vi "WS104x_NI_6501_Cntrl RF Switch.vi"(0 "SW1":bool=TRUE, 1 "NI-6051":T1={"Addr Cntrl 1"="Dev1/port0/line0", "Addr Cntrl 2"="Dev1/port0/line1", "Addr Cntrl 3"="Dev1/port0/line2", "Addr Cntrl 4"="Dev1/port0/line3"}, 5 "SW2":bool, 7 "SW3":bool, 9 "SW4":bool, 11 "error in":errorcluster) -> (15 "error out":errorcluster)   [LabVIEW 2012]
doc: "I. Description:\nThis example demonstrates how to write values to a digital output channel.\n\nII. Instructions for Running:\n1. Select the digital lines on the DAQ device to be written.\n2. Select a value to write.\nNote: The array control is sized for 8 lines, if using a different amount of lines, change the number of elements in the array to equal the number of lines chosen.\n\nIII. Block Diagram Steps:\n1. Create a Digital Output channel. Use one channel for all lines. You can alternatively use one channel for each line, but then use a different polymorphic version of the DAQmx Write VI.\n2. Call the Start VI to start the task.\n3. Write the digital Boolean array data in a loop until the user hits the stop button or an error occurs. This write VI writes a single sample of digital data on demand, so no timeout is necessary.\n4. Call the Clear Task VI to clear the Task.\n5. Use the popup dialog box to display an error or warning if any.\n\nIV. I/O Connections Overview:\nMake sure your signal output terminals match the Lines I/O Control. In this case wire the item to receive the signal to the first eight digital lines on your DAQ Device."
uses:
  <vilib>/DAQmx/create/channels.llb/DAQmx Create Channel (DO-Digital Output).vi
  <vilib>/DAQmx/write.llb/DAQmx Write (Digital Bool 1Line 1Point).vi
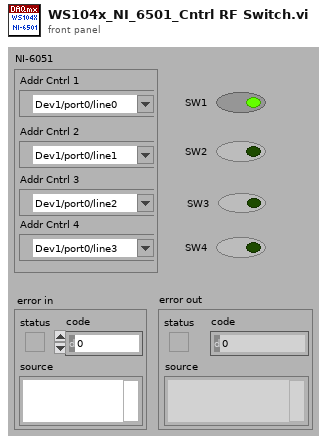
[diagram p1: front panel]
types:
  T1 = cluster{"Addr Cntrl 1":tag, "Addr Cntrl 2":tag, "Addr Cntrl 3":tag, "Addr Cntrl 4":tag}
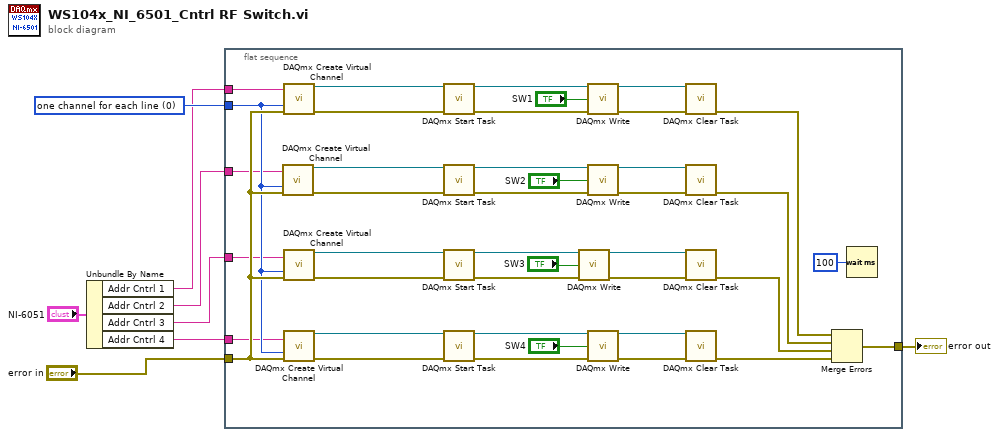
[diagram p0: block diagram]
diagram:
  w5 = 0 items=["one channel for each line", "one channel for all lines"] ("line grouping")
  n1 = Unbundle By Name("NI-6051") -> ("Addr Cntrl 1"=w4:tag, "Addr Cntrl 2"=w3:tag, "Addr Cntrl 3"=w2:tag, "Addr Cntrl 4"=w1:tag)
  n2 = flat-sequence {
    tunnel: "error in" -> [w20]
    tunnel: [w15] -> w7
    tunnel: w5 -> [w13]
    tunnel: w4 -> [w12]
    tunnel: w3 -> [w11]
    tunnel: w2 -> [w10]
    tunnel: w1 -> [w9]
    frame #0 {
      n3 = call-poly <vilib>:"DAQmx Create Virtual Channel.vi"("lines"=w11, "line grouping"=w13, "error in"=w20) -> ("task out"=w39:refnum<k21>, "error out"=w40:errorcluster)  [unwired: 11 in]
      n4 = call-poly <vilib>:"DAQmx Create Virtual Channel.vi"("lines"=w12, "line grouping"=w13, "error in"=w20) -> ("task out"=w44:refnum<k21>, "error out"=w43:errorcluster)  [unwired: 11 in]
      n5 = call-poly <vilib>:"DAQmx Create Virtual Channel.vi"("lines"=w10, "line grouping"=w13, "error in"=w20) -> ("task out"=w30:refnum<k21>, "error out"=w29:errorcluster)  [unwired: 11 in]
      n6 = call-poly <vilib>:"DAQmx Create Virtual Channel.vi"("lines"=w9, "line grouping"=w13, "error in"=w20) -> ("task out"=w25:refnum<k21>, "error out"=w26:errorcluster)  [unwired: 11 in]
      n7 = call <vilib>:"DAQmx Start Task.vi"("task/channels in"=w44, "error in"=w43) -> ("task out"=w46:refnum<k21>, "error out"=w48:errorcluster)  [unwired: 12 in]
      n8 = call <vilib>:"DAQmx Start Task.vi"("task/channels in"=w39, "error in"=w40) -> ("task out"=w37:refnum<k21>, "error out"=w35:errorcluster)  [unwired: 12 in]
      n9 = call <vilib>:"DAQmx Start Task.vi"("task/channels in"=w30, "error in"=w29) -> ("task out"=w32:refnum<k21>, "error out"=w34:errorcluster)  [unwired: 12 in]
      n10 = call <vilib>:"DAQmx Start Task.vi"("task/channels in"=w25, "error in"=w26) -> ("task out"=w23:refnum<k21>, "error out"=w21:errorcluster)  [unwired: 12 in]
      n11 = call-poly <vilib>:"DAQmx Write.vi"("task/channels in"=w32, "data"="SW3", "error in"=w34) -> ("task out"=w31:refnum<k21>, "error out"=w33:errorcluster)  [unwired: 10 in, 1 out]
      n12 = call-poly <vilib>:"DAQmx Write.vi"("task/channels in"=w46, "data"="SW1", "error in"=w48) -> ("task out"=w45:refnum<k21>, "error out"=w47:errorcluster)  [unwired: 10 in, 1 out]
      n13 = call-poly <vilib>:"DAQmx Write.vi"("task/channels in"=w37, "data"="SW2", "error in"=w35) -> ("task out"=w38:refnum<k21>, "error out"=w36:errorcluster)  [unwired: 10 in, 1 out]
      n14 = call-poly <vilib>:"DAQmx Write.vi"("task/channels in"=w23, "data"="SW4", "error in"=w21) -> ("task out"=w24:refnum<k21>, "error out"=w22:errorcluster)  [unwired: 10 in, 1 out]
      n15 = call <vilib>:"DAQmx Clear Task.vi"("task in"=w45, "error in"=w47) -> ("error out"=w19:errorcluster)  [unwired: 13 in]
      n16 = call <vilib>:"DAQmx Clear Task.vi"("task in"=w38, "error in"=w36) -> ("error out"=w18:errorcluster)  [unwired: 13 in]
      n17 = call <vilib>:"DAQmx Clear Task.vi"("task in"=w31, "error in"=w33) -> ("error out"=w17:errorcluster)  [unwired: 13 in]
      n18 = call <vilib>:"DAQmx Clear Task.vi"("task in"=w24, "error in"=w22) -> ("error out"=w16:errorcluster)  [unwired: 13 in]
      n19 = Merge Errors(w19, w18, w17, w16) -> (w15:errorcluster)
      n20 = Wait (ms)(milliseconds to wait=u32 100) -> ()  [unwired: 1 out]
    }
  }
  "error out" <- w7
